vi "Main.vi"() -> ()   [LabVIEW 2023]
uses:
  CONTROLS/States.ctl
panel:
  out "Enum":T1
  in  "stop":bool
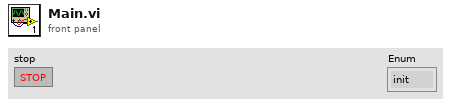
[diagram p1: front panel]
types:
  T1 = typedef "States.ctl" = enum16{"init", "read", "write", "Kundeneingabe", "Betonauswahl", "Bezahlprozess", "Rechnung", "Zudaten mit Gewichtmessung", "Stop"}
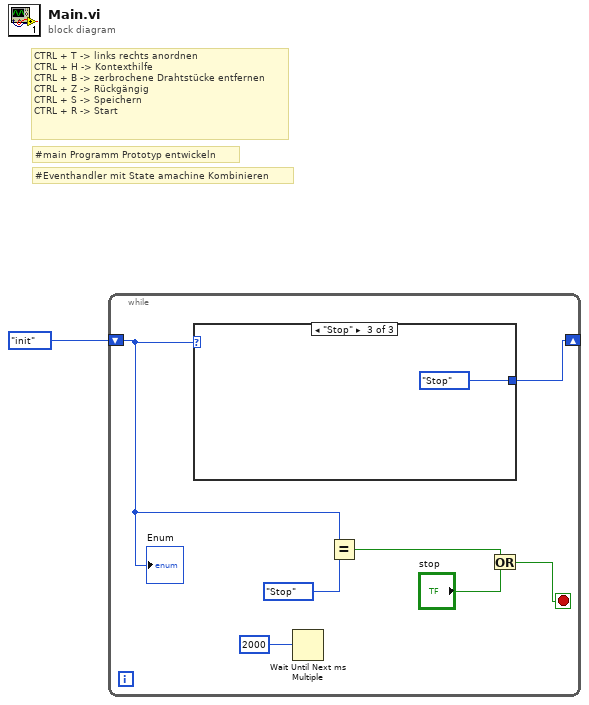
[diagram p0: block diagram]
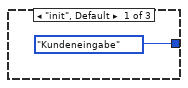
[diagram p2: hidden frame]
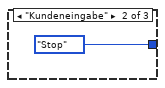
[diagram p3: hidden frame]
diagram:
  # "#Eventhandler mit State amachine Kombinieren"
  # "#main Programm Prototyp entwickeln"
  # "CTRL + T -> links rechts anordnen\nCTRL + H -> Kontexthilfe\nCTRL + B -> zerbrochene Drahtstücke entfernen\nCTRL + Z -> Rückgängig\nCTRL + S -> Speichern\nCTRL + R -> Start"
  n1 = while {
    shift-right: [w3] -> _
    shift-left: States."init" -> [w8]
    stop <- w4 stop-if-true
    n2 = case shown="\"Stop\"" w8 {
      tunnel: [States."Kundeneingabe" States."Stop" States."Stop"] -> w3
      frame "init", Default {
      }
      frame "Kundeneingabe" {
      }
      frame "Stop" {
      }
    }
    n3 = Wait Until Next ms Multiple(millisecond multiple=2000) -> ()  [unwired: 1 out]
    n4 = Equal?(x=w8, y=States."Stop") -> (x = y?=w5:bool)
    n5 = Or(x=w5, y="stop") -> (x .or. y?=w4:bool)
    "Enum" <- w8
  }
